vi "PR Set Length Of Signal.vi"(1 "Length":i32) -> (0 "LengthOfSignal":i32)   [LabVIEW 2022 SP3, in "BS6006PRPLUS.lvlib"]
doc: "The function sets the length of each signal to be acquired. The product of Length and Number, which is the input parameter of PR_SetNoAcqSignal, should be less than 262144.\n\nextern \"C\" BS6006PRPLUS_API int __cdecl PR_SetLengthOfSignal(int Length);"
uses:
  BS6006PRPLUS.lvlib
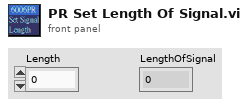
[diagram p1: front panel]
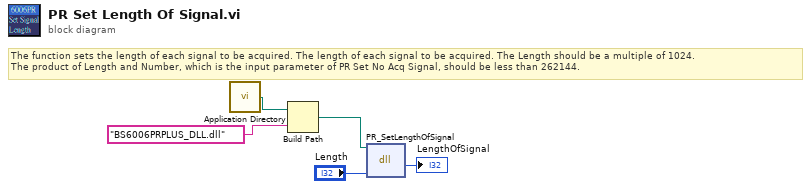
[diagram p0: block diagram]
diagram:
  # "The function sets the length of each signal to be acquired. The length of each signal to be acquired. The Length should be a multiple of 1024.\nThe product of Length and Number, which is the input parameter of PR Set No Acq Signal, should be less than 262144."
  n1 = call <vilib>:"Application Directory.vi"() -> ("Application Directory"=w3:path)
  n2 = Build Path(base path=w3, name or relative path="BS6006PRPLUS_DLL.dll") -> (appended path=w1:path)
  n3 = dll-call lib="E:/Broadsound_Program/PulserReceiver/6006PR PLUS/API/DLL/LabVIEW 15/VIs/BS6006PRPLUS_DLL.dll" fn="PR_SetLengthOfSignal"(path in=w1, "Length"="Length") -> ("return type"=→"LengthOfSignal":i32)  [unwired: 3 in, 2 out]
